vi "nirvififoEmulationP2P.vi"() -> (8 "Stream State":T1, 10 "Timeout":bool)   [LabVIEW 2017]
uses:
  <vilib>/rvi/DataTransferAndStorage/FIFO/niFpgaPeerToPeerStreamState.ctl
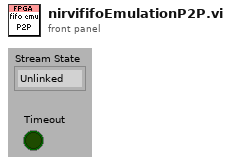
[diagram p1: front panel]
types:
  T1 = typedef "niFpgaPeerToPeerStreamState.ctl" = enum16{"Unlinked", "Disabled", "Enabled", "Flushing"}
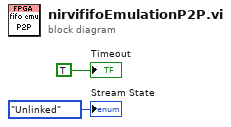
[diagram p0: block diagram]
diagram:
  "Timeout" <- TRUE ("Timeout")
  "Stream State" <- niFpgaPeerToPeerStreamState."Unlinked" ("State")
